vi "turnOffFault2.vi"   [LabVIEW 2014]
uses:
  <vilib>/DAQmx/write.llb/DAQmx Write (Digital Bool 1Line 1Point).vi
  <vilib>/DAQmx/miscellaneous.llb/DAQmx Fill In Error Info.vi
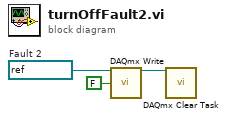
[diagram p0: block diagram]
diagram:
  w3 = refnum<k21> "DO2P1"  # Fault 2
  n1 = call-poly <vilib>:"DAQmx Write.vi"("task/channels in"=w3, "data"=FALSE) -> ("task out"=w2:refnum<k21>)  [unwired: 11 in, 2 out]
  n2 = call <vilib>:"DAQmx Clear Task.vi"("task in"=w2) -> ()  [unwired: 14 in, 1 out]
